vi "_FPGA_Driver_LTC1667_2_v1_3.vi"(8 "Clk":bool, 10 "Data in":fxp<+,14,14>) -> ()   [LabVIEW 2018]
uses:
  <vilib>/rvi/eio/common/nirviEmuTemplateMethod_errors.vi
  <vilib>/eio/EIONode/EIONode.xnode
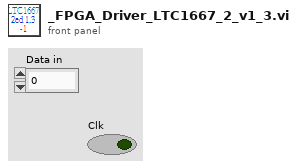
[diagram p1: front panel]
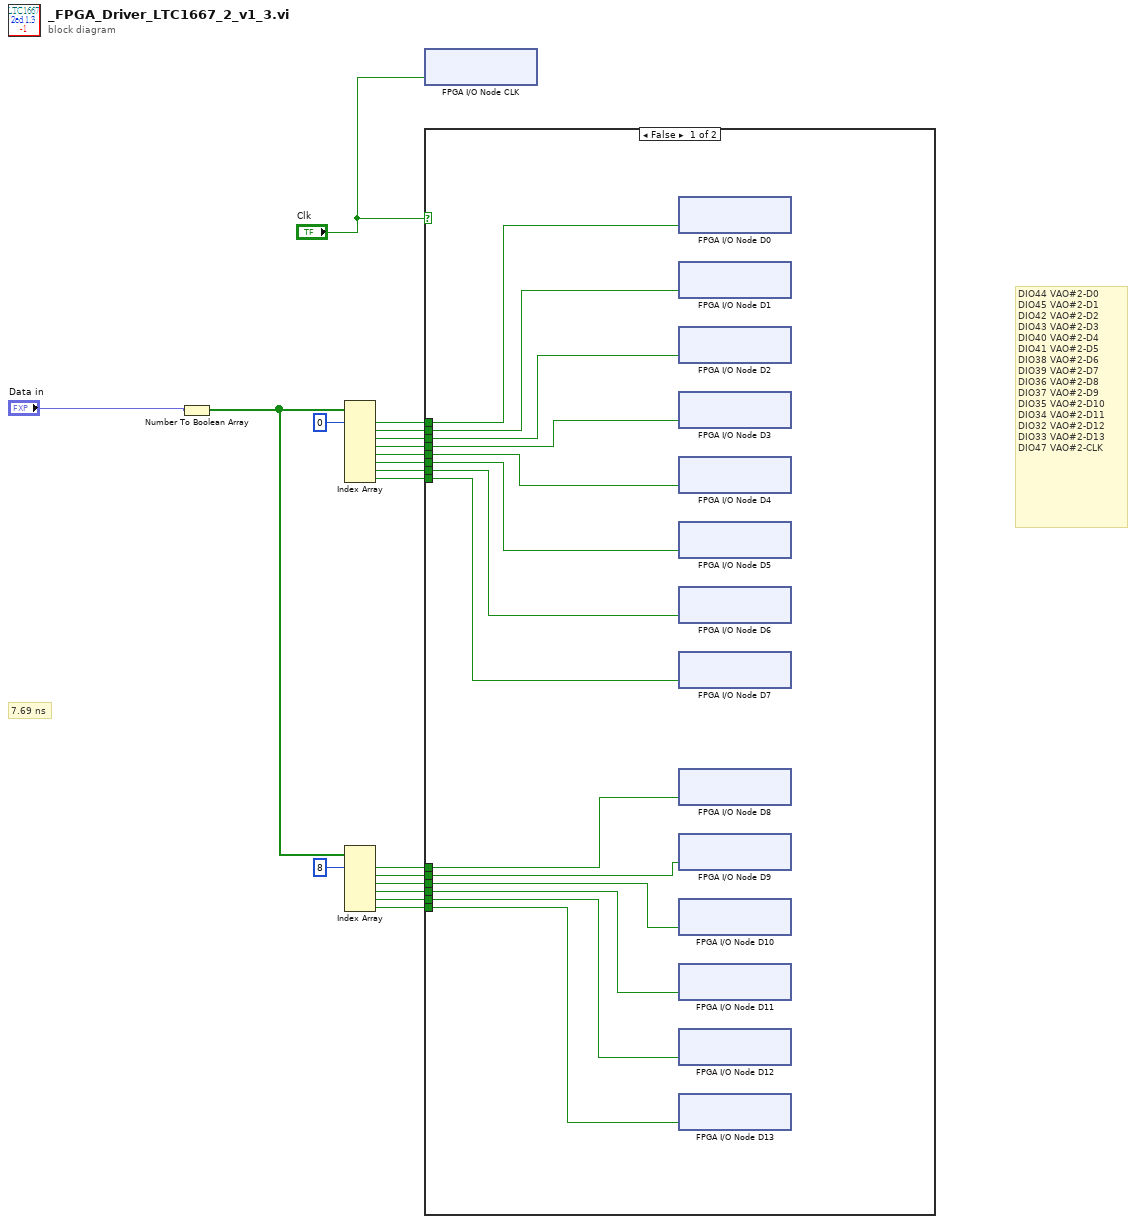
[diagram p0: block diagram]
diagram:
  # "DIO44\tVAO#2-D0\nDIO45\tVAO#2-D1\nDIO42\tVAO#2-D2\nDIO43\tVAO#2-D3\nDIO40\tVAO#2-D4\nDIO41\tVAO#2-D5\nDIO38\tVAO#2-D6\nDIO39\tVAO#2-D7\nDIO36\tVAO#2-D8\nDIO37\tVAO#2-D9\nDIO35\tVAO#2-D10\nDIO34\tVAO#2-D11\nDIO32\tVAO#2-D12\nDIO33\tVAO#2-D13\nDIO47\tVAO#2-CLK"
  # "7.69 ns"
  n1 = Number To Boolean Array(number="Data in") -> (Boolean array=w10:bool[])
  n2 = Index Array(array=w10, index #1=0 ("index")) -> (element #1=w18:bool, element #2=w17:bool, element #3=w16:bool, element #4=w15:bool, element #5=w14:bool, element #6=w13:bool, element #7=w12:bool, element #8=w11:bool)  [unwired: 7 in]
  n3 = Index Array(array=w10, index #1=8 ("index")) -> (element #1=w8:bool, element #2=w7:bool, element #3=w6:bool, element #4=w5:bool, element #5=w4:bool, element #6=w3:bool)  [unwired: 5 in]
  n4 = xnode "FPGA I/O Node CLK"("RMC/DIO47"="Clk") -> ()  [unwired: 1 in, 1 out]
  n5 = case shown="False" "Clk" {
    tunnel: w18 -> [w33 _]
    tunnel: w17 -> [w32 _]
    tunnel: w16 -> [w31 _]
    tunnel: w15 -> [w30 _]
    tunnel: w14 -> [w29 _]
    tunnel: w13 -> [w28 _]
    tunnel: w12 -> [w27 _]
    tunnel: w11 -> [w26 _]
    tunnel: w8 -> [w25 _]
    tunnel: w7 -> [w24 _]
    tunnel: w6 -> [w23 _]
    tunnel: w5 -> [w22 _]
    tunnel: w4 -> [w21 _]
    tunnel: w3 -> [w20 _]
    frame False {
      n6 = xnode "FPGA I/O Node D0"("RMC/DIO44"=w33) -> ()  [unwired: 1 in, 1 out]
      n7 = xnode "FPGA I/O Node D1"("RMC/DIO45"=w32) -> ()  [unwired: 1 in, 1 out]
      n8 = xnode "FPGA I/O Node D2"("RMC/DIO42"=w31) -> ()  [unwired: 1 in, 1 out]
      n9 = xnode "FPGA I/O Node D3"("RMC/DIO43"=w30) -> ()  [unwired: 1 in, 1 out]
      n10 = xnode "FPGA I/O Node D4"("RMC/DIO40"=w29) -> ()  [unwired: 1 in, 1 out]
      n11 = xnode "FPGA I/O Node D5"("RMC/DIO41"=w28) -> ()  [unwired: 1 in, 1 out]
      n12 = xnode "FPGA I/O Node D6"("RMC/DIO38"=w27) -> ()  [unwired: 1 in, 1 out]
      n13 = xnode "FPGA I/O Node D7"("RMC/DIO39"=w26) -> ()  [unwired: 1 in, 1 out]
      n14 = xnode "FPGA I/O Node D8"("RMC/DIO36"=w25) -> ()  [unwired: 1 in, 1 out]
      n15 = xnode "FPGA I/O Node D9"("RMC/DIO37"=w24) -> ()  [unwired: 1 in, 1 out]
      n16 = xnode "FPGA I/O Node D10"("RMC/DIO35"=w23) -> ()  [unwired: 1 in, 1 out]
      n17 = xnode "FPGA I/O Node D11"("RMC/DIO34"=w22) -> ()  [unwired: 1 in, 1 out]
      n18 = xnode "FPGA I/O Node D12"("RMC/DIO32"=w21) -> ()  [unwired: 1 in, 1 out]
      n19 = xnode "FPGA I/O Node D13"("RMC/DIO33"=w20) -> ()  [unwired: 1 in, 1 out]
    }
    frame True {
    }
  }
